vi "test_Read I16 Register Value.vi"(8 "error in (no error)":errorcluster, 11 "TestCase in":refnum<class "FPGA Register IO Tests.lvclass">=refnum) -> (0 "error out":errorcluster, 3 "TestCase out":refnum<class "FPGA Register IO Tests.lvclass">)   [LabVIEW 2026, in "FPGA Register IO Tests.lvclass"]
uses:
  FPGA Register IO Tests.lvclass
  FPGA Register IO Tests.lvclass/FPGA Register IO Tests.ctl
  APIs/FPGA Register IO/FPGA Register IO.lvlib
  <vilib>/rvi/interface/nirviCloseFPGA/nirviCloseFPGA.xnode
  <vilib>/FPGAPlugInAG/Dynamic/niLvFpga_Close_Dynamic.vi
  APIs/FPGA Register IO/Read Methods/Read Data Register/Instances/Read I16.vi
  Addon/Addon Engine/FPGA Addon Engine.lvlib
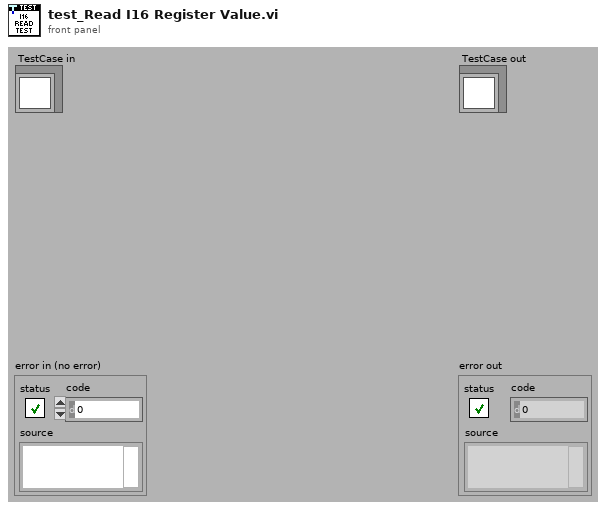
[diagram p1: front panel]
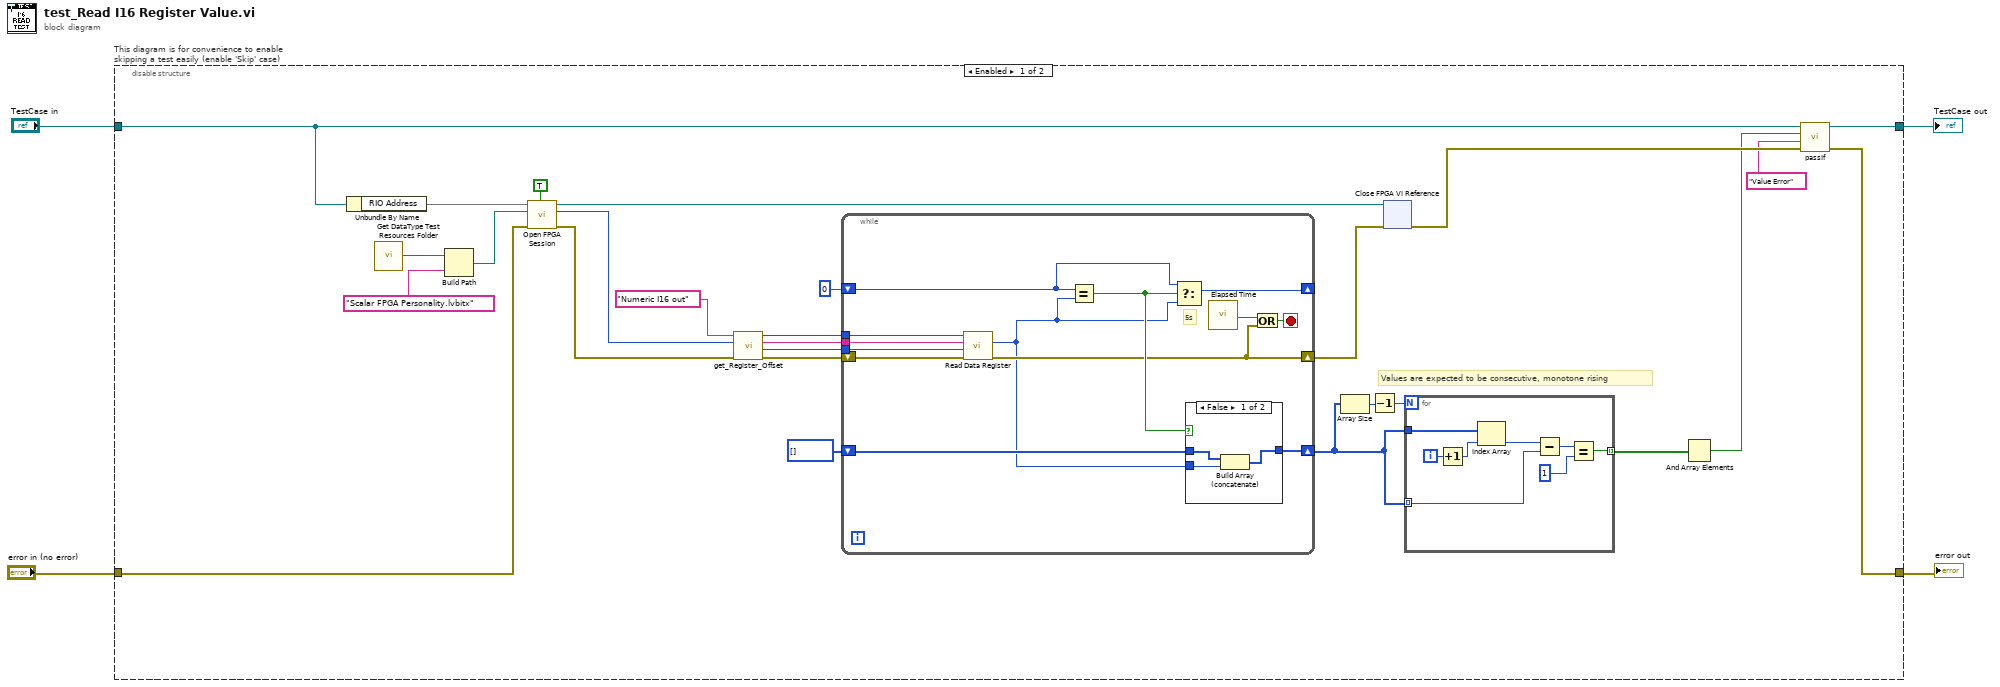
[diagram p0: block diagram]
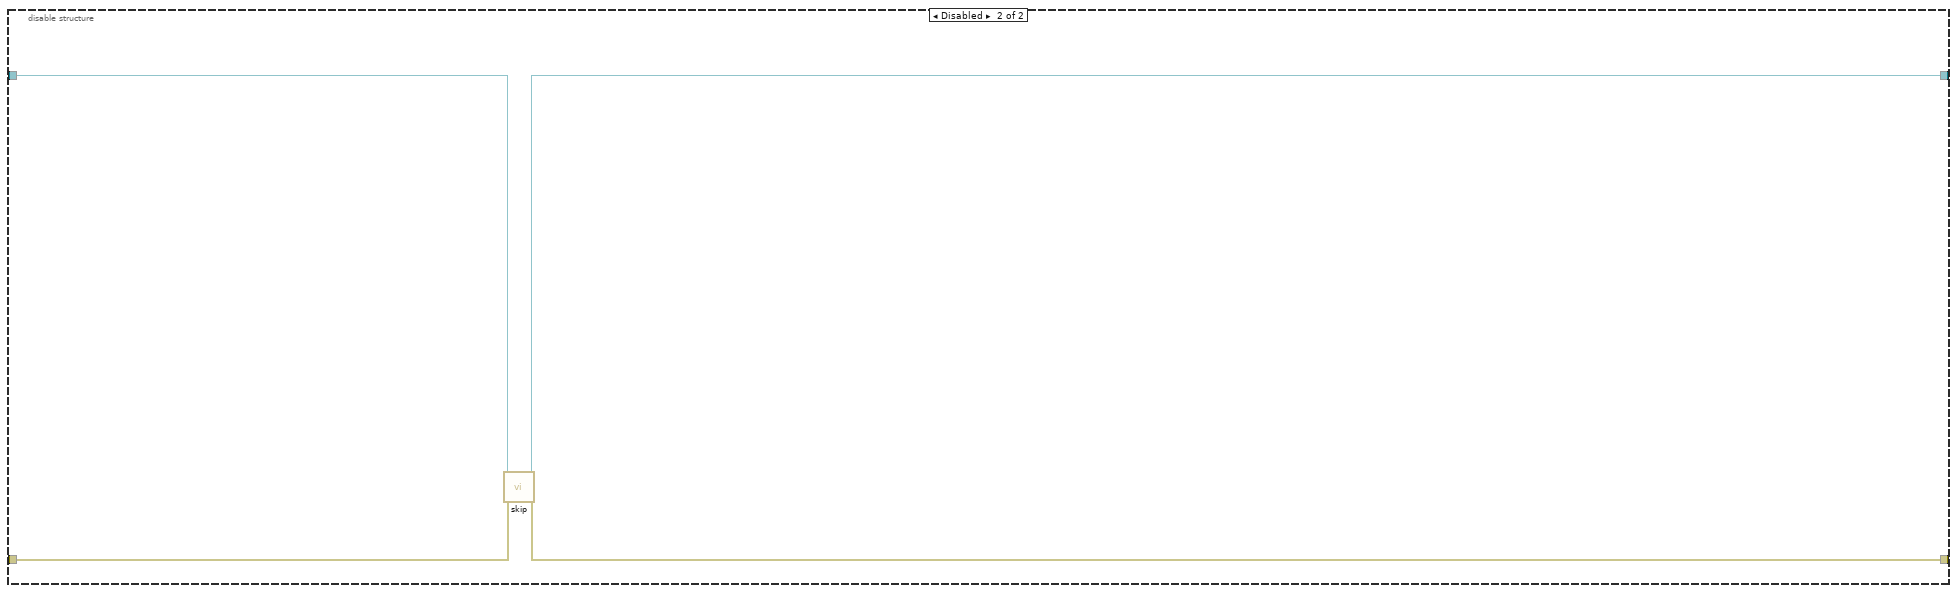
[diagram p3: hidden frame]
diagram:
  n1 = disable-structure "This diagram is for convenience to enable skipping a test easily (enable 'Skip' case)" shown="Enabled" {
    disable-tunnel: "TestCase in" -> [w18 w60]
    disable-tunnel: [w12 w58] -> w1
    disable-tunnel: [w11 w59] -> w3
    disable-tunnel: "error in (no error)" -> [w19 w57]
    frame Enabled {
      # "Values are expected to be consecutive, monotone rising"
      n2 = Unbundle By Name(w18) -> ("RIO Address"=w21)
      n3 = call "Get DataType Test Resources Folder.vi"() -> ("path"=w16:path)
      n4 = Build Path(base path=w16, name or relative path="Scalar FPGA Personality.lvbitx") -> (appended path=w20:path)
      n5 = call "Open FPGA Session.vi"("run when loaded (T)"=TRUE ("Run When Loaded (T)"), "error in"=w19, "bitfile path"=w20, "device address"=w21) -> ("error out"=w26:errorcluster, "session out"=w9:u32, "bitfile reference out"=w25:refnum<k20>)  [unwired: 5 in]
      n6 = call "get_Register_Offset.vi"("error in (no error)"=w26, "session"=w9, "Name"="Numeric I16 out" ("registerName")) -> ("error out"=w10:errorcluster, "RegisterOffset"=w5:u32, "Register Name"=w7:string, "session out"=w8:u32)  [unwired: 5 in]
      n7 = while {
        tunnel: w8 -> [w39]
        shift-right: [w35] -> w24
        shift-left: w10 -> [w38]
        shift-right: [w43] -> _
        shift-left: i16 0 ("DBL Value") -> [w44]
        shift-right: [w41] -> w27
        shift-left: i16[] [] -> [w40]
        tunnel: w7 -> [w33]
        tunnel: w5 -> [w32]
        stop <- w37 stop-if-true
        # "5s"
        n8 = call-poly "Read Data Register.vi"("error in"=w38, "RegisterOffset"=w32, "register name"=w33, "session in"=w39) -> ("error out"=w35:errorcluster, "value out"=w34:i16)  [unwired: 5 in, 1 out]
        n9 = Equal?(x=w44, y=w34) -> (x = y?=w42:bool)
        n10 = Select(t=w44, s=w42, f=w34) -> (s? t:f=w43:i16)
        n11 = case shown="False" w42 {
          tunnel: w34 -> [w47 _]
          tunnel: [w46 w48] -> w41
          tunnel: w40 -> [w45 w48]
          frame False {
            n12 = Build Array (concatenate)(w45, w47) -> (w46:i16[])
          }
          frame True {
          }
        }
        n13 = call "Elapsed Time"() -> ("Time has Elapsed"=w36:bool)  [unwired: 12 in, 7 out]
        n14 = Or(x=w36, y=w35) -> (x .or. y?=w37:bool)
      }
      n15 = Array Size(array=w27) -> (size(s)=w28:i32)
      n16 = Decrement(x=w28) -> (x-1=w29:i32)
      n17 = xnode "Close FPGA VI Reference"("FPGA VI Reference In"=w25, "error in"=w24) -> ("error out"=w17:errorcluster)
      n18 = for {
        N: w29 -> [_]
        tunnel: w27 -> [w49] mode=indexing
        tunnel: w27 -> [w56]
        tunnel: [w51] -> w30 mode=indexing
        i -> [w55]
        n19 = Increment(x=w55) -> (x+1=w54:i32)
        n20 = Index Array(array=w56, index=w54) -> (element=w50:i16)
        n21 = Subtract(x=w50, y=w49) -> (x-y=w53:i16)
        n22 = Equal?(x=w53, y=i16 1) -> (x = y?=w51:bool)
      }
      n23 = And Array Elements(Boolean array=w30) -> (logical AND=w15:bool)
      n24 = call-dynamic "passIf.vi"("error in (no error)"=w17, "message (\"\")"="Value Error" ("message (\"\")"), "pass"=w15, "TestCase in"=w18) -> ("error out"=w11:errorcluster, "TestCase out"=w12:refnum<class "FPGA Register IO Tests.lvclass">)  [unwired: 6 in]
    }
    frame Disabled {
      # "skip test result while test is under development"
      n25 = call <vilib>:"skip.vi"("error in (no error)"=w57, "TestCase in"=w60) -> ("error out"=w59:errorcluster, "TestCase out"=w58:refnum<class "FPGA Register IO Tests.lvclass">)  [unwired: 8 in]
    }
  }
  "error out" <- w3
  "TestCase out" <- w1
